vi "HSDIO_settings_to_string.vi"(8 "error in":errorcluster, 11 "HSDIO Settings":T1={"Enable HSDIO Pulses"=TRUE, "Resource Name"="PXI1Slot6", "Clock Rate"=20000000.0, "Array of Script Triggers"=[], "Pulse Generation Script"="script script1\n     wait 1\nend script", "Start Trigger"={"Wait for start trigger?"=FALSE, "source (PFI 0)"="PFI0", "edge (rising)"=12, "description"=""}, "Hardware alignment quantum\n(in samples)"=1, "Inital State"="", "Idle State"="", "Active Channels"="", "Array of Waveforms"=[], "description"=""} {"Hardware alignment quantum\n(in samples)" min=1 step=1; "Array of Script Triggers"."level" items=["High Level"=34, "Low Level"=35]; "Array of Script Triggers"."edge" items=["Rising Edge"=12, "Falling Edge"=13]; "Start Trigger"."edge (rising)" items=["Rising Edge"=12, "Falling Edge"=13]; "Clock Rate" min=0.0 max=200000000.0 format="%.2p"}) -> (0 "error out":errorcluster, 3 "resulting string":string)   [LabVIEW 2013, in "HSDIO.lvclass"]
uses:
  HSDIO.lvclass
  <instrlib>/niHSDIO/niHSDIO.llb/niHSDIO_ctl Trigger Script - trigID Values (Ring).ctl
  <instrlib>/niHSDIO/niHSDIO.llb/niHSDIO_ctl Trigger DigEdge - Edge Values (Ring).ctl
  <instrlib>/niHSDIO/niHSDIO.llb/niHSDIO_ctl Trigger Source Values (Ring).ctl
  HSDIO_settings.ctl
  <instrlib>/niHSDIO/niHSDIO.llb/niHSDIO_ctl Trigger DigLvl - Level Values (Ring).ctl
  waveform.ctl
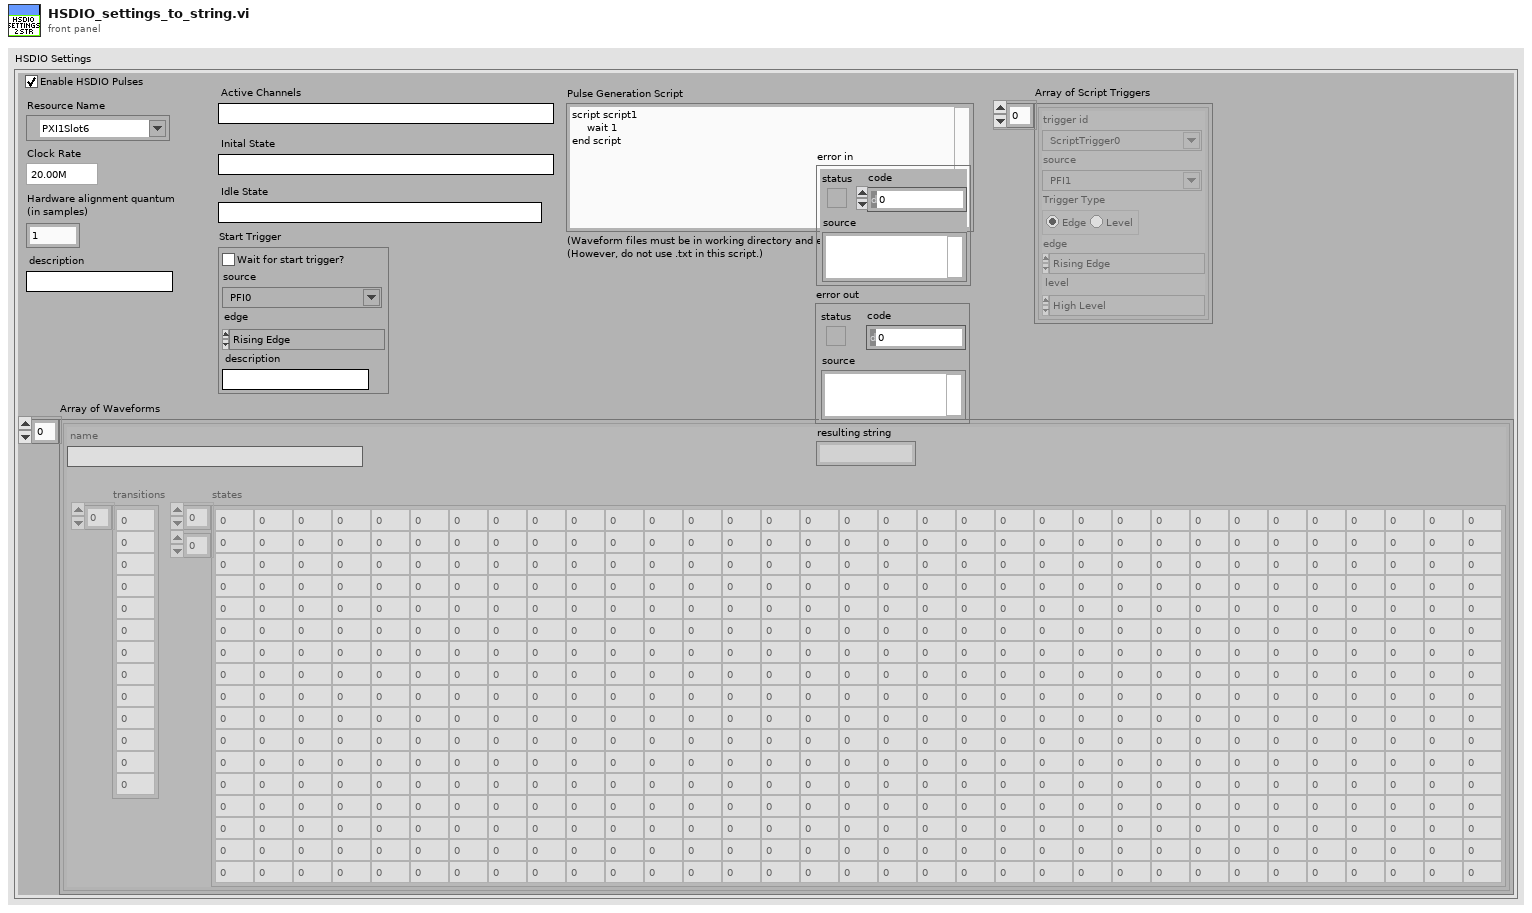
[diagram p1: front panel]
types:
  T1 = typedef "HSDIO.lvclass/HSDIO_settings.ctl" = cluster{"Enable HSDIO Pulses":bool, "Resource Name":refnum<k15>, "Clock Rate":dbl, "Array of Script Triggers":cluster{"trigger id (script trigger 0)":T2, "source (PFI 0)":T3, "Trigger Type":enum32{"Edge", "Level"}, "edge":T4, "level":T5}[], "Pulse Generation Script":string, "Start Trigger":cluster{"Wait for start trigger?":bool, "source (PFI 0)":T3, "edge (rising)":T4, "description":string}, "Hardware alignment quantum\n(in samples)":u16, "Inital State":string, "Idle State":string, "Active Channels":string, "Array of Waveforms":T6[], "description":string}
  T2 = typedef "niHSDIO_ctl Trigger Script - trigID Values (Ring).ctl" = string
  T3 = typedef "niHSDIO_ctl Trigger Source Values (Ring).ctl" = string
  T4 = typedef "niHSDIO_ctl Trigger DigEdge - Edge Values (Ring).ctl" = i32
  T5 = typedef "niHSDIO_ctl Trigger DigLvl - Level Values (Ring).ctl" = i32
  T6 = typedef "HSDIO.lvclass/waveform.ctl" = cluster{"name":string, "transitions":u32[], "states":u8[][]}
  T7 = cluster{"trigger id (script trigger 0)":T2, "source (PFI 0)":T3, "Trigger Type":enum32{"Edge", "Level"}, "edge":T4, "level":T5}[]
  T8 = cluster{"Wait for start trigger?":bool, "source (PFI 0)":T3, "edge (rising)":T4, "description":string}
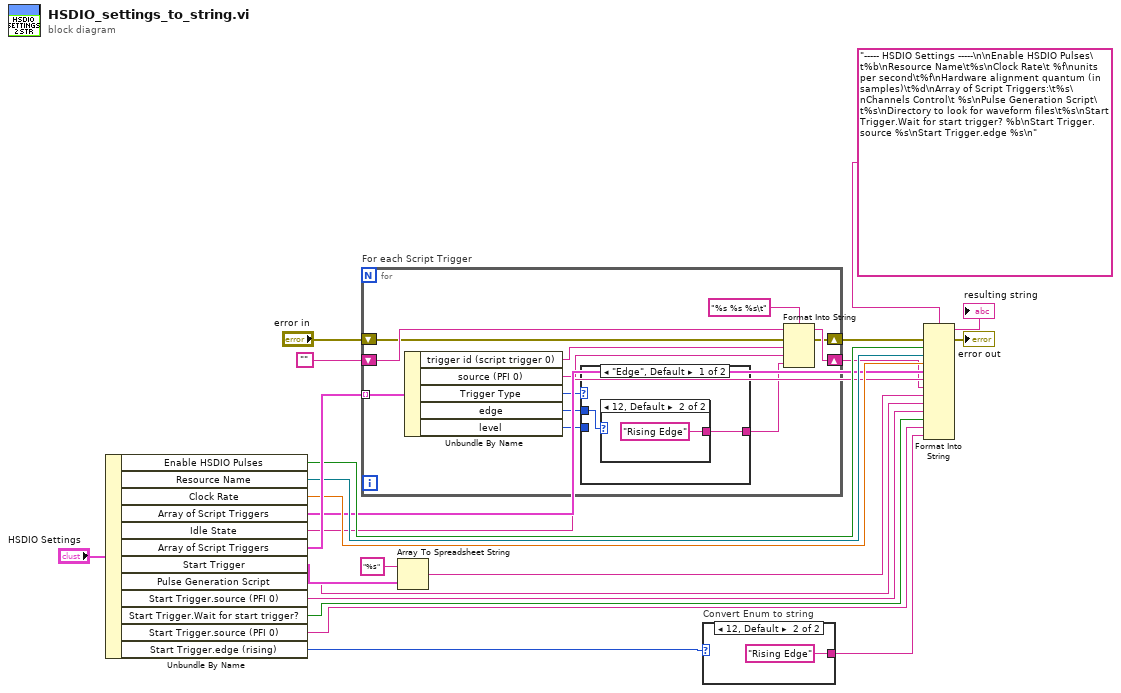
[diagram p0: block diagram]
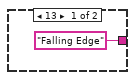
[diagram p2: hidden frame]
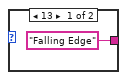
[diagram p3: hidden frame]
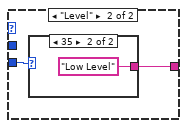
[diagram p4: hidden frame]
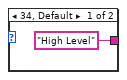
[diagram p5: hidden frame]
diagram:
  n1 = Unbundle By Name("HSDIO Settings") -> ("Enable HSDIO Pulses"=w19:bool, "Resource Name"=w16:refnum<k15>, "Clock Rate"=w15:dbl, "Array of Script Triggers"=w14:T7, "Idle State"=w13:string, "Array of Script Triggers"=w21:T7, "Start Trigger"=w11:T8, "Pulse Generation Script"=w8:string, "Start Trigger.source (PFI 0)"=w7:T3, "Start Trigger.Wait for start trigger?"=w6:bool, "Start Trigger.source (PFI 0)"=w5:T3, "Start Trigger.edge (rising)"=w4:T4)
  n2 = for "For each Script Trigger" {
    tunnel: w21 -> [w35] mode=indexing
    shift-right: [w26] -> w12
    shift-left: "" -> [w27]
    shift-right: [w24] -> w17
    shift-left: "error in" -> [w25]
    n3 = Unbundle By Name(w35) -> ("trigger id (script trigger 0)"=w34:T2, "source (PFI 0)"=w33:T3, "Trigger Type"=w31:enum32{"Edge", "Level"}, "edge"=w30:T4, "level"=w29:T5)
    n4 = case shown="\"Edge\", Default" w31 {
      tunnel: w30 -> [w37 _]
      tunnel: [w36 w40] -> w28
      tunnel: w29 -> [_ w41]
      frame "Edge", Default {
        n5 = case shown="12, Default" w37 {
          tunnel: ["Falling Edge" "Rising Edge"] -> w36
          frame 13 {
          }
          frame 12, Default {
          }
        }
      }
      frame "Level" {
        n6 = case shown="35" w41 {
          tunnel: ["High Level" "Low Level"] -> w40
          frame 34, Default {
          }
          frame 35 {
          }
        }
      }
    }
    n7 = Format Into String(format string="%s %s %s\t", initial string=w27, error in=w25, w34, w33, w28) -> (resulting string=w26:string, error out=w24:errorcluster)
  }
  n8 = Array To Spreadsheet String(array=w11, 3:"%s" ("format string")) -> (spreadsheet string=w10:string)  [unwired: 1 in]
  n9 = case "Convert Enum to string" shown="12, Default" w4 {
    tunnel: ["Falling Edge" "Rising Edge"] -> w3
    frame 13 {
    }
    frame 12, Default {
    }
  }
  n10 = Format Into String(format string="----- HSDIO Settings -----\n\nEnable HSDIO Pulses\t%b\nResource Name\t%s\nClock Rate\t %f\nunits per second\t%f\nHardware alignment quantum (in samples)\t%d\nArray of Script Triggers:\t%s\nChannels Control\t %s\nPulse Generation Script\t%s\nDirectory to look for waveform files\t%s\nStart Trigger.Wait for start trigger? %b\nStart Trigger.source %s\nStart Trigger.edge %s\n", error in=w17, w19, w16, w15, w14, w13, w12, w10, w8, w7, w6, w5, w3) -> (resulting string=→"resulting string":string, error out=→"error out":errorcluster)  [unwired: 1 in]
